vi "Select Mouse PPL.vi"() -> (3 "selected path":path, 5 "cancelled":bool)   [LabVIEW 2020, in "App.lvlib" / "MazeUI.lvclass"]
uses:
  MazeUI.lvclass
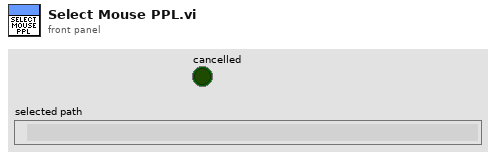
[diagram p1: front panel]
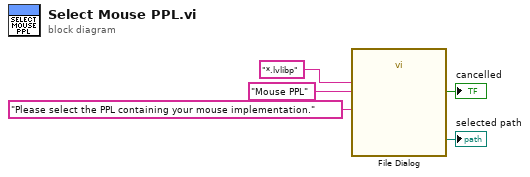
[diagram p0: block diagram]
diagram:
  n1 = call "File Dialog"("prompt"="Please select the PPL containing your mouse implementation.", "pattern (all files)"="*.lvlibp", "pattern label"="Mouse PPL") -> ("selected path"=→"selected path":path, "cancelled"=→"cancelled":bool)  [unwired: 9 in, 2 out]
